vi "host-C-Experimental-1 (1).vi"() -> (0 "K(Indicator)":fxp<+/-,64,32>=1.52587890625e-05, 1 "degree":dbl=0.1952712924057206, 2 "Nominal Freq":fxp<+/-,64,32>=0.494873046875)   [LabVIEW 2012]
uses:
  <vilib>/rvi/interface/nirviReadWriteControl/nirviReadWriteControl.xnode
  <vilib>/rvi/interface/nirviMethod/nirviMethod.xnode
  <vilib>/rvi/interface/nirviCloseFPGA/nirviCloseFPGA.xnode
  <vilib>/rvi/interface/nirviOpenFPGA/nirviOpenFPGA.xnode
  SB130-XPS/Documents/FPGA-project-apporach-retraction/FPGA Bitfiles/Apporach-Retract_FPGATarget_LIAFPGA3a-PDTest_L-X5ia9B-g4.lvbitx
  LIA_FPGA3a-PD Test.vi
  <vilib>/Utility/file.llb/Write To Spreadsheet File (DBL).vi
  <vilib>/rvi/errors/niLvFpgaMergeErrorWithErrorCode.vi
  <vilib>/FPGAPlugInAG/Dynamic/niLvFpga_Close_Dynamic.vi
  <vilib>/FPGAPlugInAG/Dynamic/niLvFpga_ReadFifo_Dynamic.vi
panel:
  out "Corrected Frequency":fxp<+/-,64,32>
  out "Angular Frequency":fxp<+/-,64,32>
  out "Z":fxp<+/-,64,32>
  in  "Nominal Frequency 2":fxp<+/-,64,32>
  in  "PID Error":fxp<+/-,64,32>
  in  "VCO Constant 2":fxp<+/-,64,10>
  out "Waveform Chart 2":i32[](graph)
  out "Waveform Chart":i32[](graph)
  in  "Number of Elements":i32
  in  "Proportional Gain":fxp<+/-,64,32>
  in  "Integral Gain":fxp<+/-,64,32>
  out "P+I Error":fxp<+/-,64,32>
  out "PID Input Error":dbl
  out "Phase (Degree) Shift":fxp<+/-,64,32>
  out "Numeric":fxp<+/-,64,32>
  out "For Proportional":fxp<+/-,64,32>
  in  "DAQ Acquisition Rate":i32
  in  "Wait":i32
  in  "Frequency Modulation Start":bool
  in  "Path 5":path
  in  "name-file 11":string="approach-15a"
  out "String 11":string
  in  "Path 7":path
  in  "name-file 9":string="approach-15a"
  out "String 9":string
  in  "Path 4":path
  in  "name-file 4":string="approach-15a"
  out "String 4":string
  in  "Path 3":path
  in  "name-file 3":string="approach-15a"
  out "String 3":string
  in  "Path 2":path
  in  "name-file 2":string="approach-15a"
  out "String 2":string
  in  "Data Collector":bool
  out "String":string
  in  "name-file":string="approach-15a"
  in  "Path":path
  out "Standardized nominal freq":dbl
  in  "Delta Nominal Frequency":dbl
  out "Ref":i32
  out "Sig":i32
  out "Sin":dbl(graph)
  out "Phase":dbl
  out "Ze Output":dbl=2.3841857910156248e-12
  out "The Decs":dbl=7.8125e-09
  out "LSB Weight":dbl=0.00030517578125
  in  "K":fxp<+,16,0>=1.52587890625e-05
  in  "nominal freq 2":fxp<+,16,0>=0.494873046875
  out "x*y":dbl=0.015
  in  "stop 2":bool
  out "3rd stages":i32=1
  out "3rd decimation":i32=977
  out "1st decimation":i32=1
  out "2nd decimation":i32=128
  in  "Time Constant [s]":dbl=2.5 min=0.0 step=0.0001 format="%.2f"
  in  "Filter Rolloff":enum16{"20 dB", "40 dB", "60 dB", "80 dB"}(ring)
  out "Actual Sampling Frequency":dbl=200000.0
  in  "input range of 9205":dbl=10.0
  in  "Sampling Frequency":dbl=200000.0 min=1000.0 max=250000.0
  in  "stop":bool
  out "r":dbl(graph)=0.5098420210496609
  out "y":dbl=0.0017376029872894286
  out "x":dbl=0.5098390600609779
  out "f":dbl(graph)=31000.332441180944
  in  "dec2":i16=1
  in  "nominal freq":dbl=30000.0 min=500.0 max=125000.0
  in  "dec1":i16=1000
  in  "stages":i8=1 min=1 max=2
  in  "decimation":i16=1000
  # "Sampling Frequency"
  # "CIC First Decimation"
  # "MA Stages"
  # "CIC Second Decimation"
  # "PLL Nominal Frequency"
  # "MA Decimation"
  # "PLL Frequency Output"
  # "LIA Output"
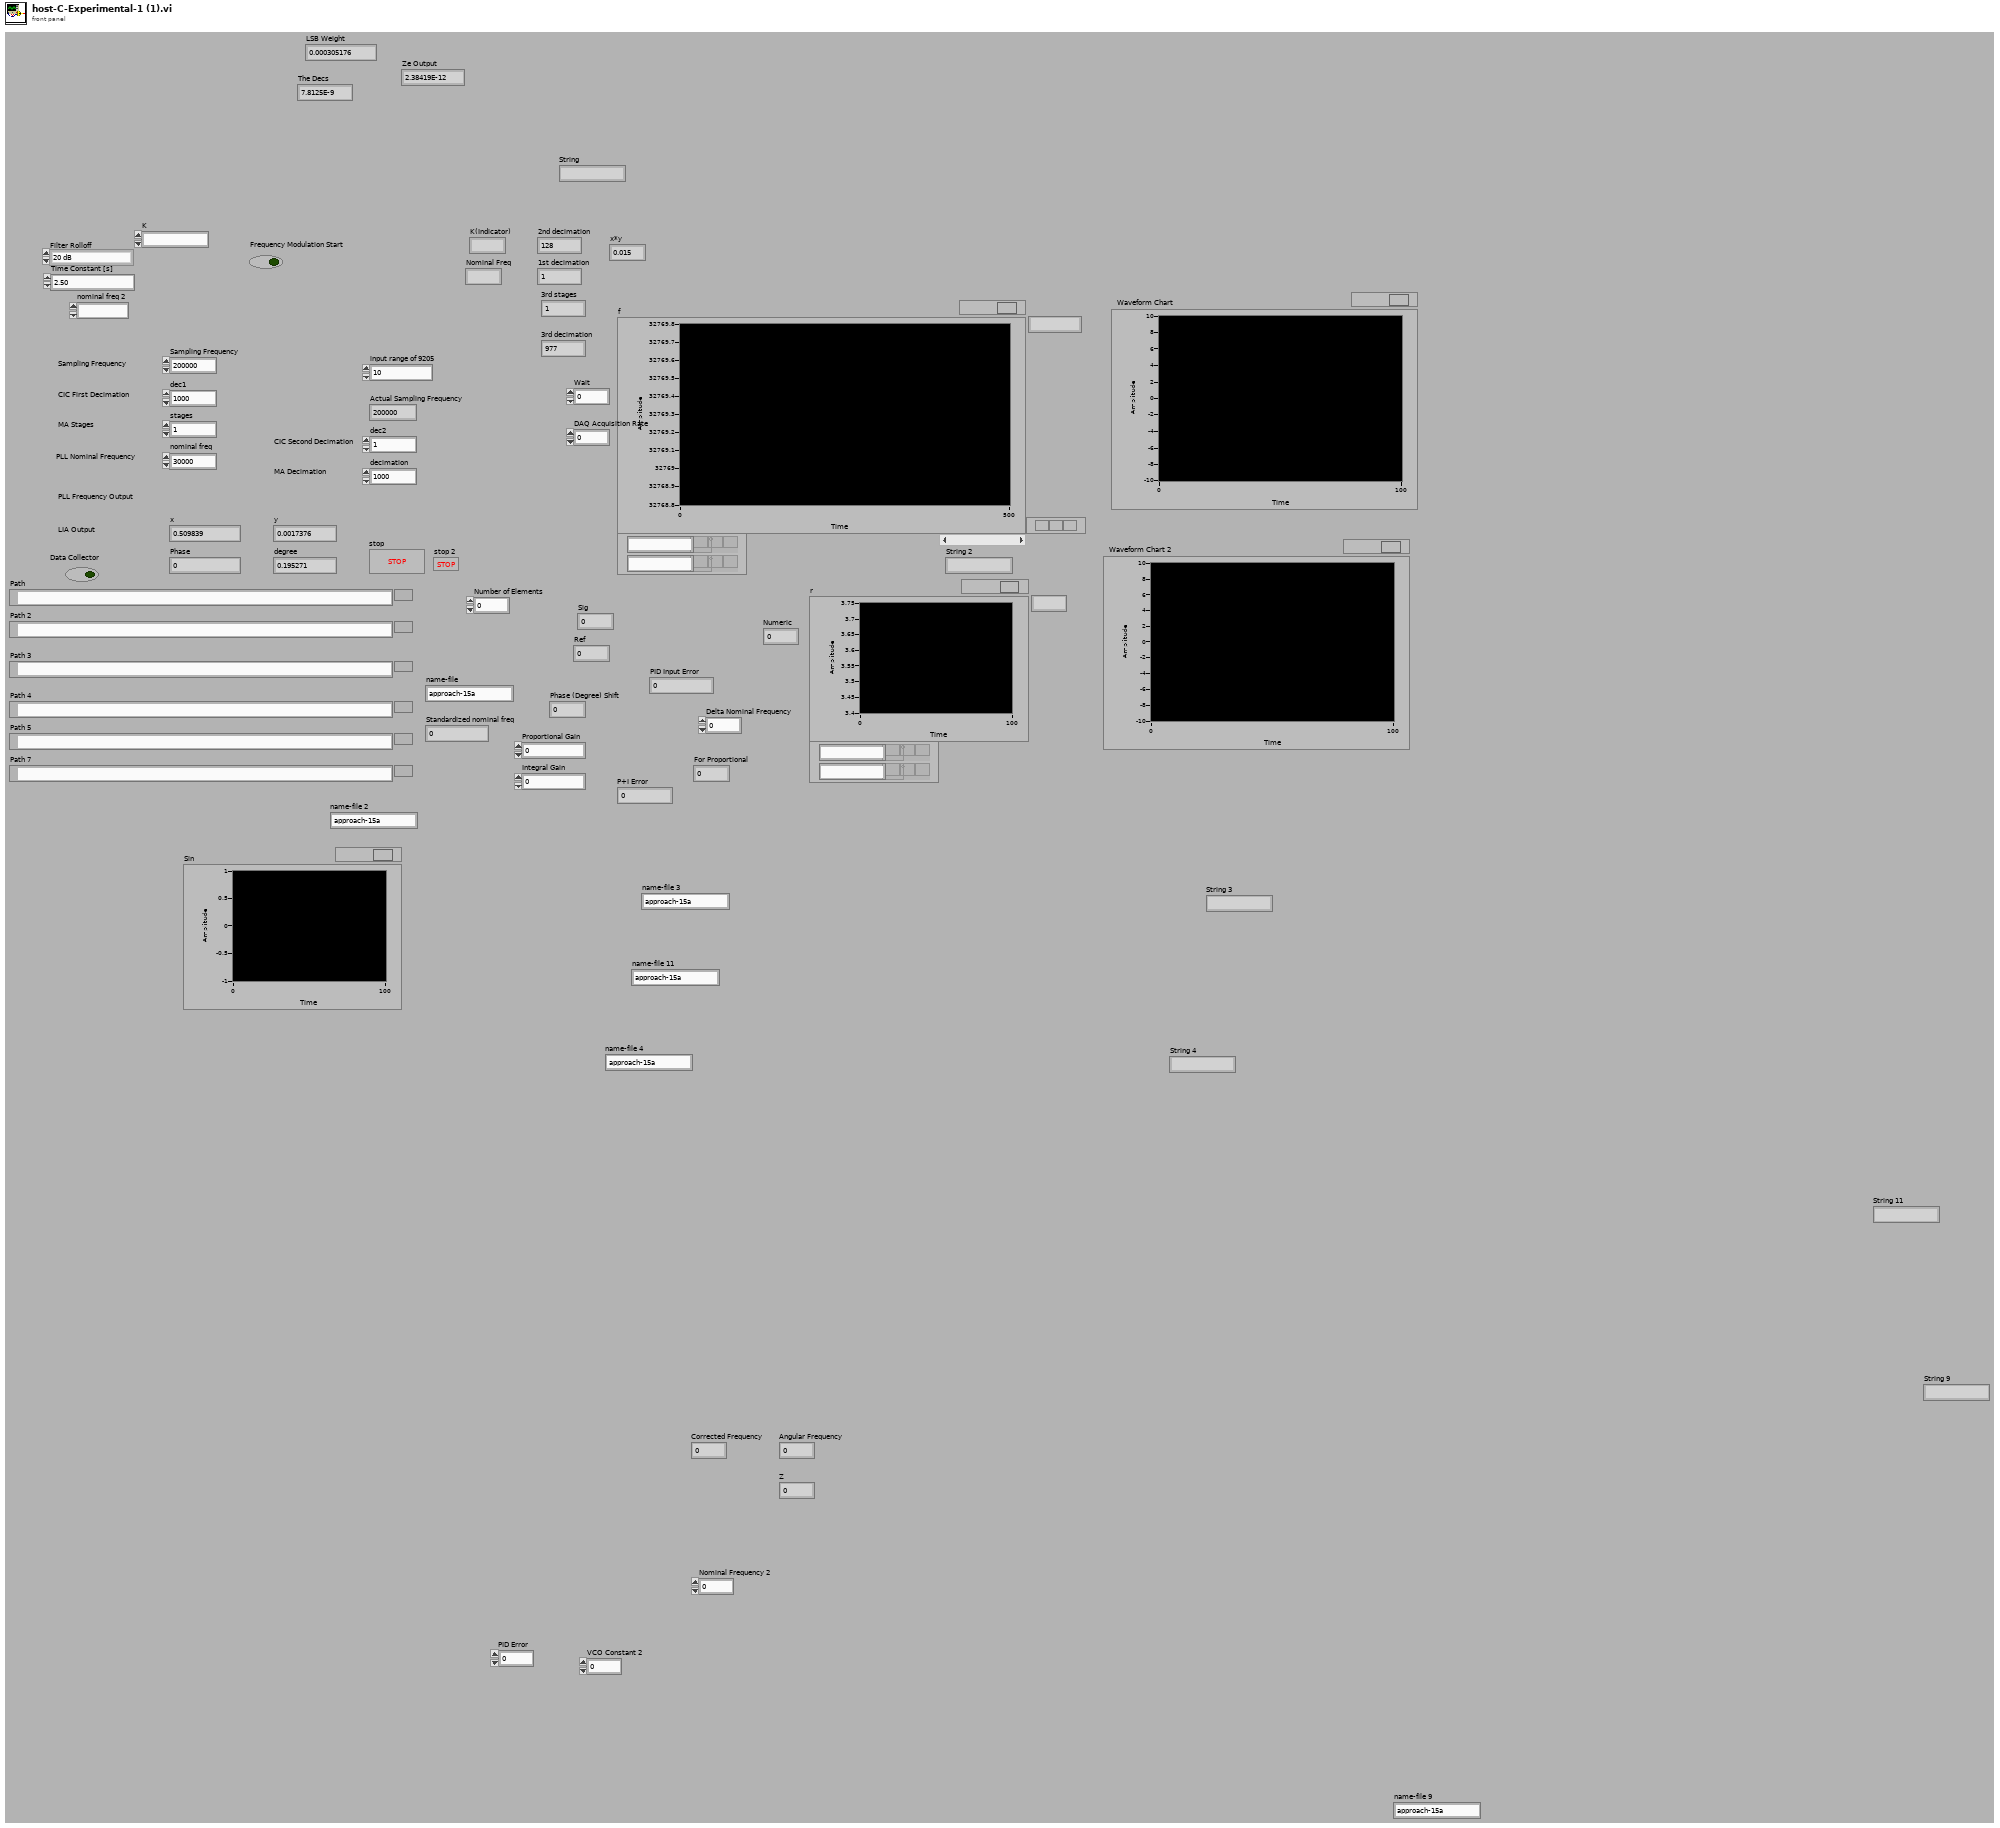
[diagram p1: front panel]
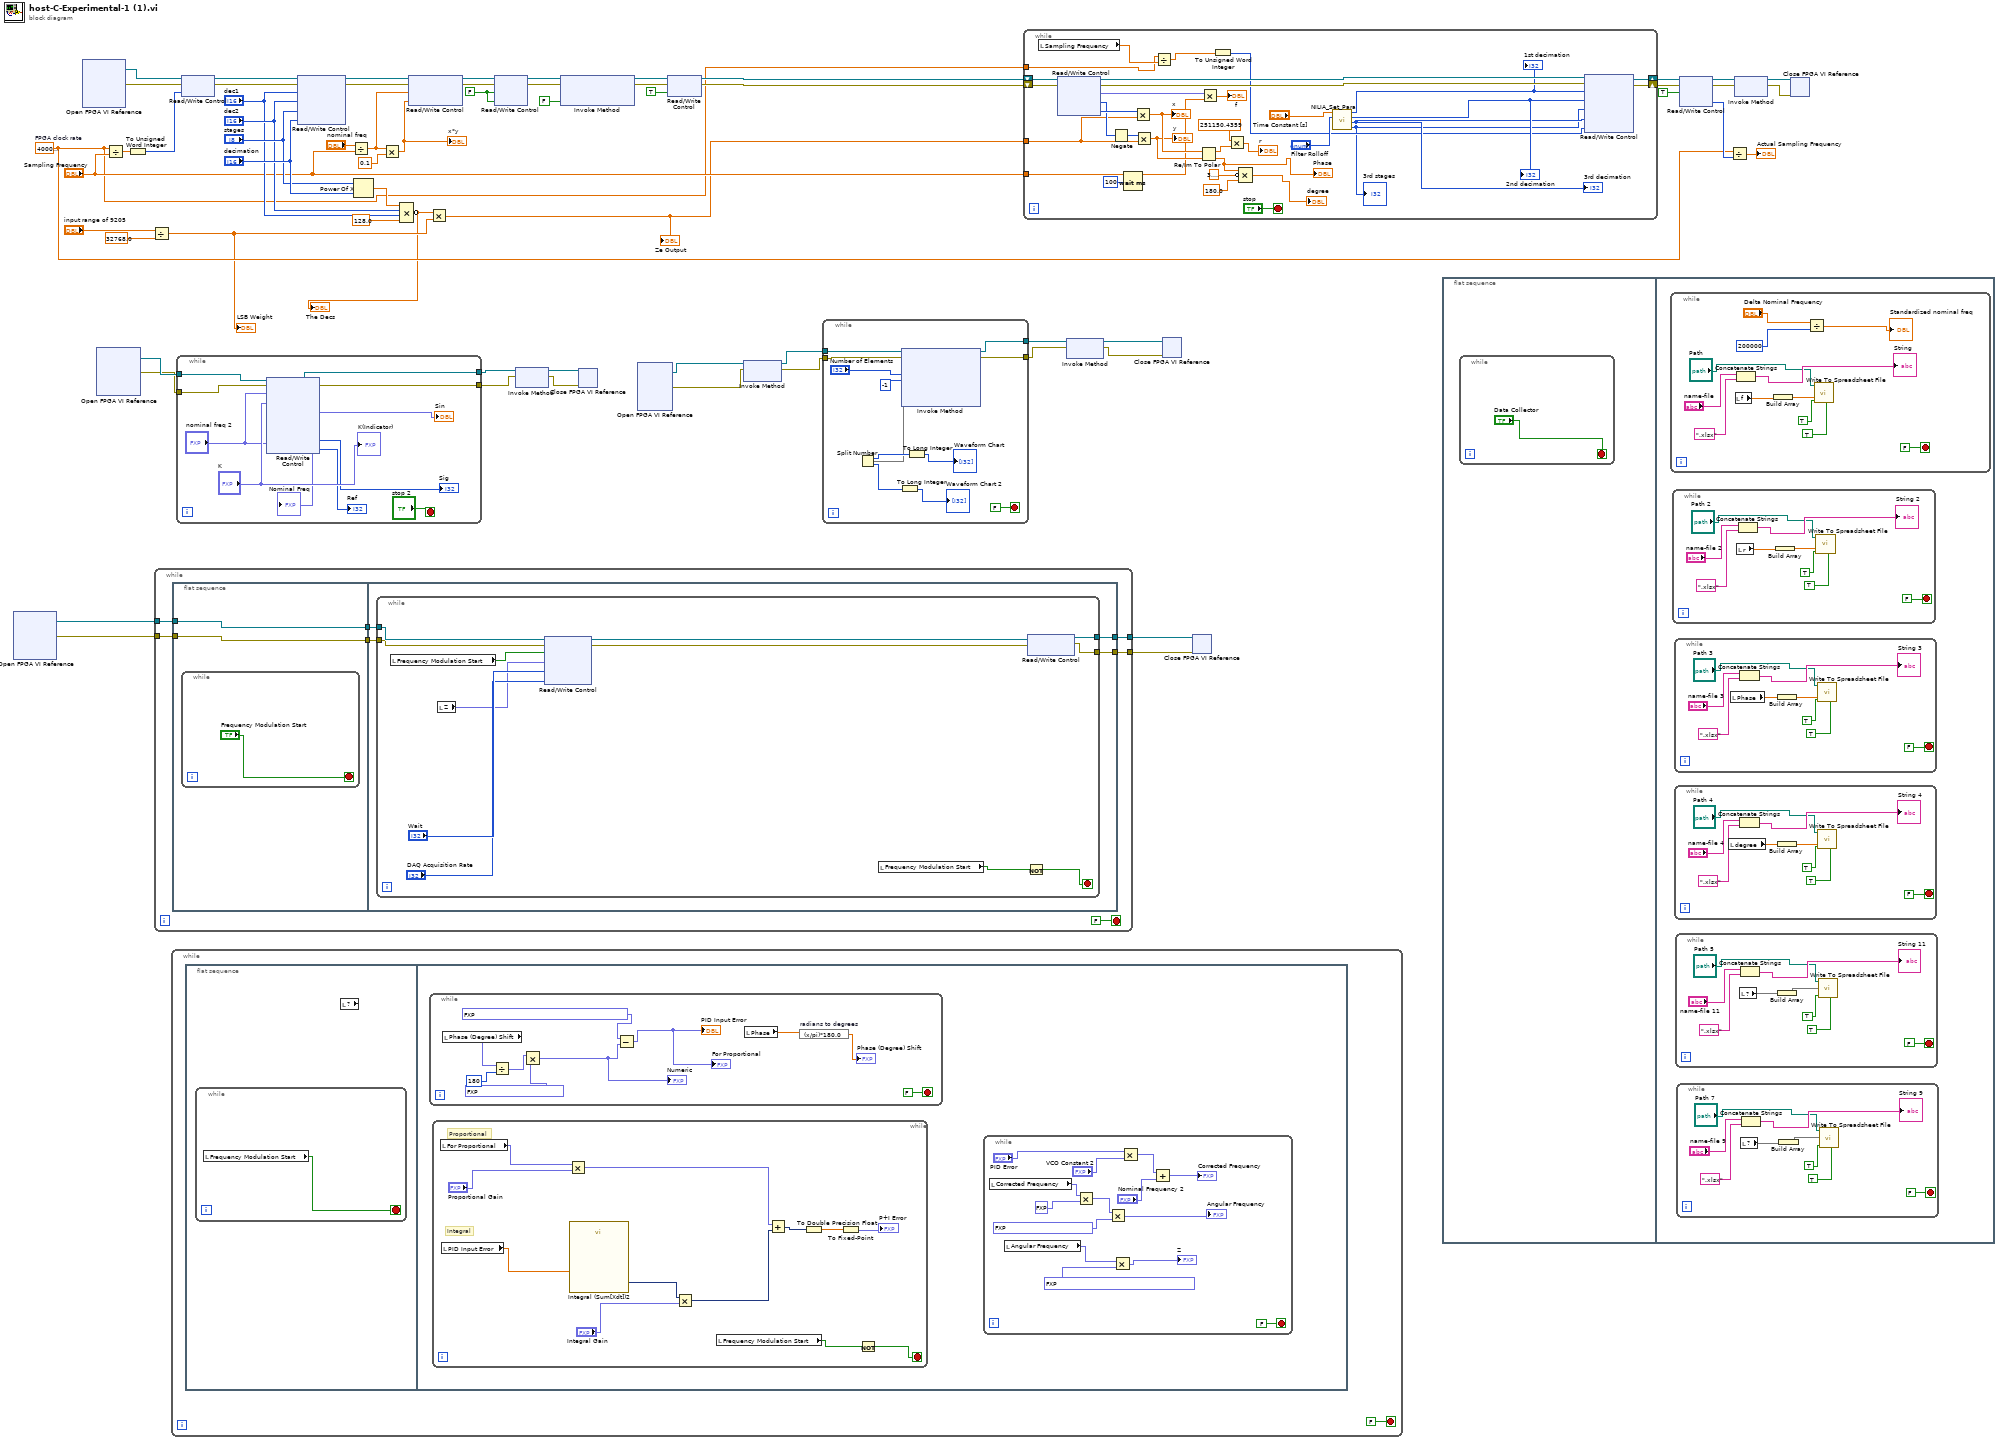
[diagram p0: block diagram]
diagram:
  w23 = 40000000.0  # FPGA clock rate
  w42 = FALSE ("start")
  n1 = xnode "Open FPGA VI Reference"() -> ("FPGA VI Reference Out"=w10:refnum<k20>, "error out"=w9:errorcluster)  [unwired: 2 in]
  n2 = xnode "Open FPGA VI Reference"() -> ("FPGA VI Reference Out"=w29:refnum<k20>, "error out"=w28:errorcluster)  [unwired: 2 in]
  n3 = xnode "Open FPGA VI Reference"() -> ("FPGA VI Reference Out"=w22:refnum<k20>, "error out"=w21:errorcluster)  [unwired: 2 in]
  n4 = Divide(x=w23, y="Sampling Frequency") -> (x/y=w35:dbl)
  n5 = To Unsigned Word Integer(number=w35) -> (unsigned 16bit integer=w34:u16)
  n6 = Divide(x="input range of 9205", y=32768.0) -> (x/y=w15:dbl)
  "LSB Weight" <- w15
  n7 = while {
    tunnel: [w69] -> w12
    tunnel: [w68] -> w11
    tunnel: w10 -> [w66]
    tunnel: w9 -> [w64]
    stop <- FALSE stop-if-true
    n8 = flat-sequence {
      tunnel: [w72] -> w67
      tunnel: w66 -> [w72]
      tunnel: [w71] -> w65
      tunnel: w64 -> [w71]
      tunnel: [w77] -> w69
      tunnel: [w76] -> w68
      tunnel: w67 -> [w75]
      tunnel: w65 -> [w74]
      frame #0 {
        n9 = while {
          stop <- "Frequency Modulation Start" stop-if-true
        }
      }
      frame #1 {
        n10 = while {
          tunnel: [w87] -> w77
          tunnel: [w86] -> w76
          tunnel: w75 -> [w85]
          tunnel: w74 -> [w84]
          stop <- w88 stop-if-true
          n11 = local read "Frequency Modulation Start"() -> (w79:bool)
          n12 = local read "Z"() -> (w78:fxp<+/-,64,32>)
          n13 = xnode "Read/Write Control"("FPGA VI Reference In"=w85, "error in"=w84, "Unselected"=w79, "Unselected"=w78, "Unselected"="Wait", "Unselected"="DAQ Acquisition Rate") -> ("FPGA VI Reference Out"=w82:refnum<k20>, "error out"=w83:errorcluster)
          n14 = local read "Frequency Modulation Start"() -> (w89:bool)
          n15 = Not(x=w89) -> (.not. x?=w88:bool)
          n16 = xnode "Read/Write Control"("FPGA VI Reference In"=w82, "error in"=w83) -> ("FPGA VI Reference Out"=w87:refnum<k20>, "error out"=w86:errorcluster)  [unwired: 1 in]
        }
      }
    }
  }
  n17 = while {
    stop <- FALSE stop-if-true
    n18 = flat-sequence {
      frame #0 {
        n19 = while {
          stop <- w91 stop-if-true
          n20 = local read "Frequency Modulation Start"() -> (w91:bool)
        }
        n21 = local read item#-1() -> ()  [unwired: 1 out]
      }
      frame #1 {
        n22 = while {
          stop <- FALSE stop-if-true
          n23 = local read "Phase (Degree) Shift"() -> (w106:fxp<+/-,64,32>)
          n24 = Divide(x=w106, y=i16 180) -> (x/y=w114:fxp<+/-,64,33>)
          n25 = Multiply(x=w114, y=fxp<+,30,2> 3.1415926814079285) -> (x*y=w113:fxp<+/-,64,35>)
          "Numeric" <- w113
          n26 = Subtract(x=fxp<+,50,1> 1.5707963199999995, y=w113) -> (x-y=→"PID Input Error" →"For Proportional":fxp<+/-,64,36>)
          n27 = local read "Phase"() -> (w108:dbl)
          n28 = expression code="(x/pi)*180.0" "radians to degrees"(w108) -> (→"Phase (Degree) Shift":dbl)
        }
        n29 = while {
          stop <- w116 stop-if-true
          # "Integral"
          # "Proportional"
          n30 = local read "For Proportional"() -> (w127:fxp<+/-,64,32>)
          n31 = local read "PID Input Error"() -> (w125:dbl)
          n32 = Multiply(x=w127, y="Proportional Gain") -> (x*y=w122:fxp<+/-,64,64>)
          n33 = call "Integral (Sum[Xdt])2"("Signals"=w125) -> ("Result"=w124:dynamicdata)  [unwired: 5 in, 1 out]
          n34 = Multiply(x=w124, y="Integral Gain") -> (x*y=w121:dynamicdata)
          n35 = local read "Frequency Modulation Start"() -> (w117:bool)
          n36 = Add(x=w122, y=w121) -> (x+y=w120:dynamicdata)
          n37 = To Double Precision Float(number=w120) -> (double precision float=w119:dbl)
          n38 = To Fixed-Point(number=w119) -> (fixed-point=→"P+I Error":fxp<+/-,32,16>)  [unwired: 1 in]
          n39 = Not(x=w117) -> (.not. x?=w116:bool)
        }
        n40 = while {
          stop <- FALSE stop-if-true
          n41 = local read "Corrected Frequency"() -> (w97:fxp<+/-,64,32>)
          n42 = local read "Angular Frequency"() -> (w102:fxp<+/-,64,32>)
          n43 = Multiply(x=w97, y=fxp<+,1,2> 2.0) -> (x*y=w100:fxp<+/-,64,33>)
          n44 = Multiply(x=w100, y=fxp<+,30,2> 3.1415926814079285) -> (x*y=→"Angular Frequency":fxp<+/-,64,35>)
          n45 = Multiply(x=w102, y=fxp<+,46,7> 0.0010000000002037268) -> (x*y=→"Z":fxp<+/-,64,39>)
          n46 = Multiply(x="PID Error", y="VCO Constant 2") -> (x*y=w94:fxp<+/-,64,42>)
          n47 = Add(x=w94, y="Nominal Frequency 2") -> (x+y=→"Corrected Frequency":fxp<+/-,64,43>)
        }
      }
    }
  }
  n48 = while {
    tunnel: w22 -> [w136]
    tunnel: w21 -> [w135]
    tunnel: [w134] -> w20
    tunnel: [w133] -> w19
    stop <- "stop 2" stop-if-true
    n49 = xnode "Read/Write Control"("FPGA VI Reference In"=w136, "error in"=w135, "nominal freq"="nominal freq 2", "K"="K") -> ("FPGA VI Reference Out"=w134:refnum<k20>, "error out"=w133:errorcluster, "Sin"=→"Sin":fxp<+/-,14,2>, "sig"=→"Sig":i16, "ref"=→"Ref":i16)  [unwired: 2 out]
    "K(Indicator)" <- "K"
    "Nominal Freq" <- "nominal freq 2"
  }
  n50 = xnode "Read/Write Control"("FPGA VI Reference In"=w29, "error in"=w28, "Period"=w34) -> ("FPGA VI Reference Out"=w37:refnum<k20>, "error out"=w36:errorcluster)
  n51 = xnode "Read/Write Control"("FPGA VI Reference In"=w37, "error in"=w36, "dec1"="dec1", "dec2"="dec2", "stages"="stages", "decimation"="decimation") -> ("FPGA VI Reference Out"=w63:refnum<k20>, "error out"=w62:errorcluster)
  n52 = Divide(x="nominal freq", y="Sampling Frequency") -> (x/y=w31:dbl)
  n53 = Power Of X(1:"decimation", 2:"stages") -> (0:w58:dbl)
  n54 = Multiply(x=w31, y=0.1) -> (x*y=w16:dbl)
  "x*y" <- w16
  n55 = Compound Arithmetic op=MULTIPLY(w58, "dec2", "dec1", 128.0) -> (invert w14:dbl)
  "The Decs" <- w14
  n56 = xnode "Read/Write Control"("FPGA VI Reference In"=w63, "error in"=w62, "nominal freq"=w31, "K"=w16) -> ("FPGA VI Reference Out"=w46:refnum<k20>, "error out"=w45:errorcluster)
  n57 = Multiply(x=w14, y=w15) -> (x*y=w13:dbl)
  "Ze Output" <- w13
  n58 = xnode "Read/Write Control"("FPGA VI Reference In"=w46, "error in"=w45, "start"=w42, "stop"=w42) -> ("FPGA VI Reference Out"=w44:refnum<k20>, "error out"=w43:errorcluster)
  n59 = xnode "Invoke Method"("FPGA VI Reference In"=w20, "error in"=w19) -> ("FPGA VI Reference Out"=w18:refnum<k20>, "error out"=w17:errorcluster)
  n60 = xnode "Invoke Method"("FPGA VI Reference In"=w44, "error in"=w43, "Wait Until Done (F)"=FALSE) -> ("FPGA VI Reference Out"=w51:refnum<k20>, "error out"=w49:errorcluster)
  n61 = xnode "Close FPGA VI Reference"("FPGA VI Reference In"=w18, "error in"=w17) -> ()  [unwired: 1 out]
  n62 = xnode "Open FPGA VI Reference"() -> ("FPGA VI Reference Out"=w8:refnum<k20>, "error out"=w7:errorcluster)  [unwired: 2 in]
  n63 = xnode "Read/Write Control"("FPGA VI Reference In"=w51, "error in"=w49, "start"=TRUE) -> ("FPGA VI Reference Out"=w50:refnum<k20>, "error out"=w48:errorcluster)
  n64 = xnode "Invoke Method"("FPGA VI Reference In"=w8, "error in"=w7) -> ("FPGA VI Reference Out"=w6:refnum<k20>, "error out"=w5:errorcluster)
  n65 = while {
    tunnel: w6 -> [w141]
    tunnel: w5 -> [w140]
    tunnel: [w139] -> w2
    tunnel: [w138] -> w1
    stop <- FALSE stop-if-true
    n66 = xnode "Invoke Method"("FPGA VI Reference In"=w141, "error in"=w140, "Number of Elements"="Number of Elements", "Timeout (ms)"=-1) -> ("FPGA VI Reference Out"=w139:refnum<k20>, "error out"=w138:errorcluster, "Data"=w144:void[])  [unwired: 1 out]
    n67 = Split Number(x=w144) -> (hi(x)=w146:u16[], lo(x)=w145:u16[])
    n68 = To Long Integer(number=w145) -> (32bit integer=→"Waveform Chart 2":i32[])
    n69 = To Long Integer(number=w146) -> (32bit integer=→"Waveform Chart":i32[])
  }
  n70 = while {
    shift-right: [w166] -> w54
    shift-left: w50 -> [w181]
    shift-right: [w165] -> w53
    shift-left: w48 -> [w180]
    tunnel: w13 -> [w177]
    tunnel: "Sampling Frequency" -> [w169]
    tunnel: w23 -> [w158]
    stop <- "stop" stop-if-true
    n71 = local read "Sampling Frequency"() -> (w159:dbl)
    n72 = xnode "Read/Write Control"("FPGA VI Reference In"=w181, "error in"=w180) -> ("FPGA VI Reference Out"=w166:refnum<k20>, "error out"=w165:errorcluster, "f"=w170:fxp<+/-,32,0>, "channelQ"=w178:i64, "channelI"=w179:i64)
    n73 = Negate(x=w178) -> (-x=w167:i64)
    n74 = Wait (ms)(milliseconds to wait=u32 100) -> ()  [unwired: 1 out]
    n75 = Multiply(x=w179, y=w177) -> (x*y=w176:dbl)
    "x" <- w176
    n76 = Multiply(x=w167, y=w177) -> (x*y=w175:dbl)
    "y" <- w175
    n77 = Divide(x=w158, y=w159) -> (x/y=w157:dbl)
    n78 = Re/Im To Polar(2:w175, 3:w176) -> (0:w150:dbl, 1:w153:dbl)
    "Phase" <- w150
    n79 = Multiply(x=w170, y=w169) -> (x*y=→"f":dbl)
    n80 = To Unsigned Word Integer(number=w157) -> (unsigned 16bit integer=w156:u16)
    n81 = Multiply(x=251150.4359, y=w153) -> (x*y=→"r":dbl)
    n82 = Compound Arithmetic op=MULTIPLY(w150, invert 3.141592653589793, 180.0 ("value")) -> (→"degree":dbl)
    n83 = call "NILIA_Set_Para.vi"("rolloff"="Filter Rolloff", "TC [sec]"="Time Constant [s]") -> ("3rd stages"=w155:i32, "3rd decimation"=w160:i32, "2nd decimation"=w161:i32, "1st decimation"=w162:i32)  [unwired: 5 in, 1 out]
    "2nd decimation" <- w161
    "1st decimation" <- w162
    "3rd decimation" <- w160
    "3rd stages" <- w155
    n84 = xnode "Read/Write Control"("FPGA VI Reference In"=w166, "error in"=w165, "dec1"=w162, "dec2"=w161, "stages"=w155, "decimation"=w160, "Period"=w156) -> ()  [unwired: 2 out]
  }
  n85 = xnode "Invoke Method"("FPGA VI Reference In"=w2, "error in"=w1) -> ("FPGA VI Reference Out"=w4:refnum<k20>, "error out"=w3:errorcluster)
  n86 = xnode "Close FPGA VI Reference"("FPGA VI Reference In"=w4, "error in"=w3) -> ()  [unwired: 1 out]
  n87 = xnode "Close FPGA VI Reference"("FPGA VI Reference In"=w12, "error in"=w11) -> ()  [unwired: 1 out]
  n88 = flat-sequence {
    frame #0 {
      n89 = while {
        stop <- "Data Collector" stop-if-true
      }
    }
    frame #1 {
      n90 = while {
        stop <- FALSE stop-if-true
        n91 = local read "f"() -> (w235:dbl)
        n92 = Concatenate Strings("name-file", ".xlsx") -> (→"String":string)
        n93 = Build Array(w235) -> (w234:dbl[])
        n94 = Divide(x="Delta Nominal Frequency", y=200000) -> (x/y=→"Standardized nominal freq":dbl)
        n95 = call-poly <vilib>:"Write To Spreadsheet File.vi"("transpose? (no:F)"=TRUE, "append to file? (new file:F)"=TRUE, "1D data"=w234, "file path (dialog if empty)"="Path") -> ()  [unwired: 4 in, 1 out]
      }
      n96 = while {
        stop <- FALSE stop-if-true
        n97 = local read "r"() -> (w226:dbl)
        n98 = Concatenate Strings("name-file 2", ".xlsx") -> (→"String 2":string)
        n99 = Build Array(w226) -> (w225:dbl[])
        n100 = call-poly <vilib>:"Write To Spreadsheet File.vi"("transpose? (no:F)"=TRUE, "append to file? (new file:F)"=TRUE, "1D data"=w225, "file path (dialog if empty)"="Path 2") -> ()  [unwired: 4 in, 1 out]
      }
      n101 = while {
        stop <- FALSE stop-if-true
        n102 = local read "Phase"() -> (w217:dbl)
        n103 = Concatenate Strings("name-file 3", ".xlsx") -> (→"String 3":string)
        n104 = Build Array(w217) -> (w216:dbl[])
        n105 = call-poly <vilib>:"Write To Spreadsheet File.vi"("transpose? (no:F)"=TRUE, "append to file? (new file:F)"=TRUE, "1D data"=w216, "file path (dialog if empty)"="Path 3") -> ()  [unwired: 4 in, 1 out]
      }
      n106 = while {
        stop <- FALSE stop-if-true
        n107 = local read "degree"() -> (w208:dbl)
        n108 = Concatenate Strings("name-file 4", ".xlsx") -> (→"String 4":string)
        n109 = Build Array(w208) -> (w207:dbl[])
        n110 = call-poly <vilib>:"Write To Spreadsheet File.vi"("transpose? (no:F)"=TRUE, "append to file? (new file:F)"=TRUE, "1D data"=w207, "file path (dialog if empty)"="Path 4") -> ()  [unwired: 4 in, 1 out]
      }
      n111 = while {
        stop <- FALSE stop-if-true
        n112 = local read item#-1() -> (w190)
        n113 = Concatenate Strings("name-file 11", ".xlsx") -> (→"String 11":string)
        n114 = Build Array(w190) -> (w189:void[])
        n115 = call-poly <vilib>:"Write To Spreadsheet File.vi"("transpose? (no:F)"=TRUE, "append to file? (new file:F)"=TRUE, "1D data"=w189, "file path (dialog if empty)"="Path 5") -> ()  [unwired: 4 in, 1 out]
      }
      n116 = while {
        stop <- FALSE stop-if-true
        n117 = local read item#-1() -> (w199)
        n118 = Concatenate Strings("name-file 9", ".xlsx") -> (→"String 9":string)
        n119 = Build Array(w199) -> (w198:void[])
        n120 = call-poly <vilib>:"Write To Spreadsheet File.vi"("transpose? (no:F)"=TRUE, "append to file? (new file:F)"=TRUE, "1D data"=w198, "file path (dialog if empty)"="Path 7") -> ()  [unwired: 4 in, 1 out]
      }
    }
  }
  n121 = xnode "Read/Write Control"("FPGA VI Reference In"=w54, "error in"=w53, "stop"=TRUE) -> ("FPGA VI Reference Out"=w41:refnum<k20>, "error out"=w40:errorcluster, "ticks"=w25:u16)
  n122 = Divide(x=w23, y=w25) -> (x/y=→"Actual Sampling Frequency":dbl)
  n123 = xnode "Invoke Method"("FPGA VI Reference In"=w41, "error in"=w40) -> ("FPGA VI Reference Out"=w39:refnum<k20>, "error out"=w38:errorcluster)
  n124 = xnode "Close FPGA VI Reference"("FPGA VI Reference In"=w39, "error in"=w38) -> ()  [unwired: 1 out]
